vi "Calculate Target Pose.vi"(6 "Distance to target (in)":dbl=36.0, 8 "Robot Calibration Cluster":T1={"Camera Height on robot (in)"=34.5, "Camera Angle on the robot (deg)"=28.3, "Camera FOV Top to Bottom View Angle (deg)"=0.946, "Target size (in)"=6.5, "Distance to front of bumper (in)"=9.75, "Focal Length (mm)"=10.0} {"Focal Length (mm)" format="%#_13g"; "Distance to front of bumper (in)" format="%#_13g"; "Target size (in)" format="%#_13g"; "Camera FOV Top to Bottom View Angle (deg)" format="%#_13g"; "Camera Angle on the robot (deg)" format="%#_13g"; "Camera Height on robot (in)" format="%#_13g"}, 9 "Camera Resolution":T2={"Camera Resolution W (pixels)"=800.0, "Camera Resolution H (pixels)"=600.0}, 10 "Corners":cluster{"X":dbl, "Y":dbl}[](array[cluster])=[{"X"=420.0, "Y"=290.0}, {"X"=480.0, "Y"=290.0}, {"X"=420.0, "Y"=350.0}, {"X"=480.0, "Y"=350.0}], 11 "Target Center":cluster{"X":dbl, "Y":dbl}) -> (1 "Target Roll (deg)":dbl, 2 "Target Pitch (deg)":dbl, 3 "Target Yaw (deg)":dbl)   [LabVIEW 2023]
uses:
  Camera Info.ctl
panel:
  out "3D Position (inches)":cluster{"X":dbl, "Y":dbl, "Z":dbl}
  out "Z'":dbl
  out "Y'":dbl
  out "Z (in)":dbl=36.0
  out "Y (in)":dbl
  out "X (in)":dbl
  out "Theta y (deg)":dbl
  out "Theta x (deg)":dbl
  out "Focal length in pixels":dbl
  out "Sensor height (mm)":dbl
  out "Sensor width (mm)":dbl
  in  "Sensor pixel size (µm)":dbl=3.0
  # "Bottom Left"
  # "Bottom Right"
  # "Top Right"
  # "Top Left"
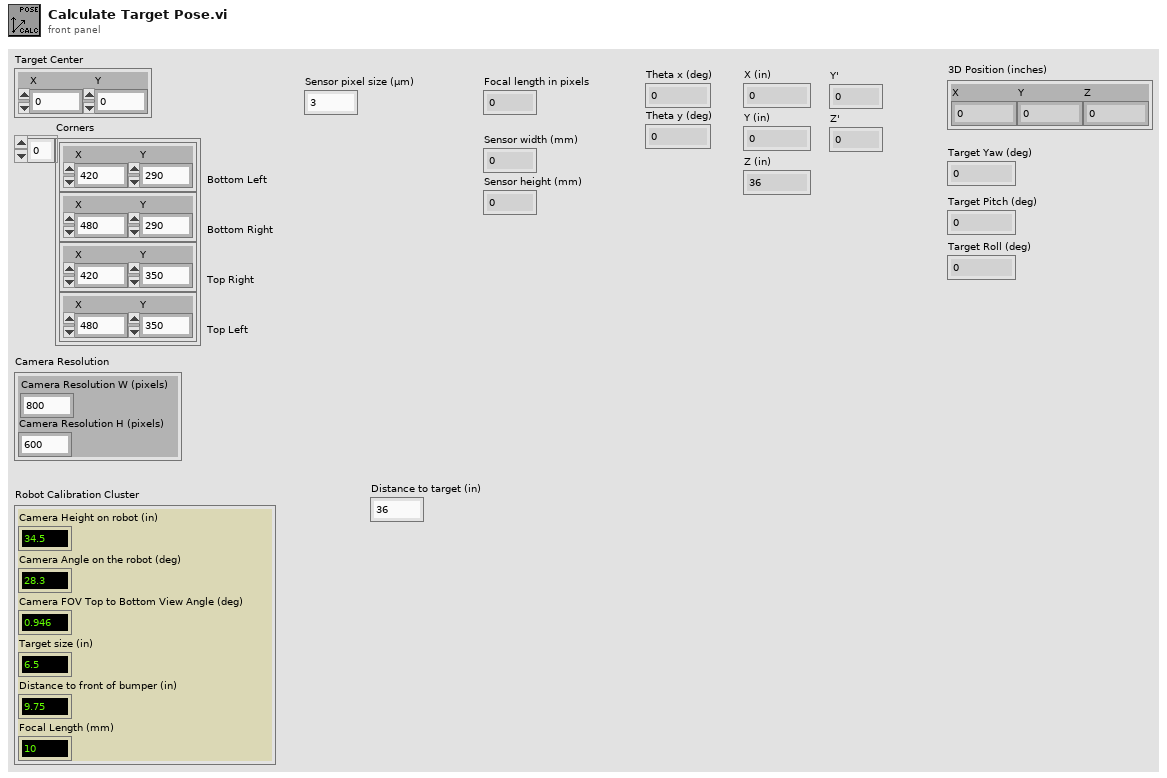
[diagram p1: front panel]
types:
  T1 = typedef "Camera Info.ctl" = cluster{"Camera Height on robot (in)":dbl, "Camera Angle on the robot (deg)":dbl, "Camera FOV Top to Bottom View Angle (deg)":dbl, "Target size (in)":dbl, "Distance to front of bumper (in)":dbl, "Focal Length (mm)":dbl}
  T2 = cluster{"Camera Resolution W (pixels)":dbl, "Camera Resolution H (pixels)":dbl}
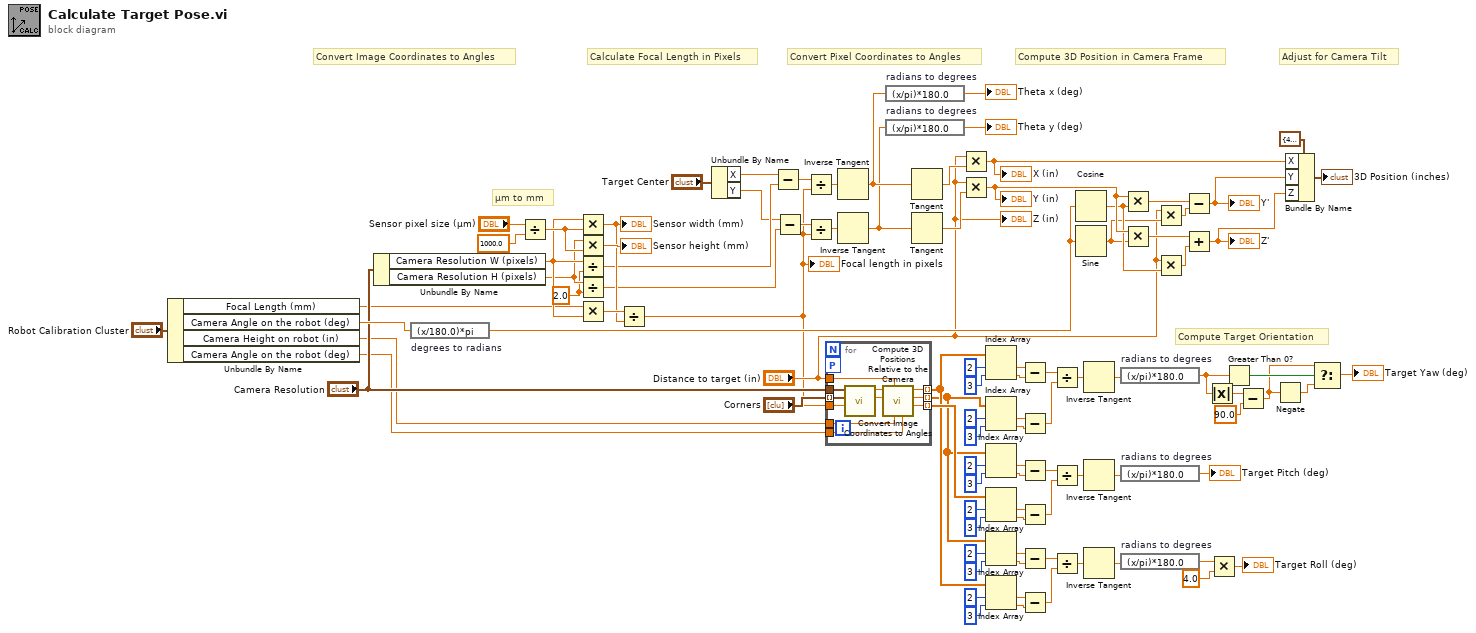
[diagram p0: block diagram]
diagram:
  w65 = 2.0 ("y")
  # "Compute Target Orientation"
  # "Adjust for Camera Tilt"
  # "Compute 3D Position in Camera Frame"
  # "Convert Pixel Coordinates to Angles"
  # "Calculate Focal Length in Pixels"
  # "µm to mm"
  # "Convert Image Coordinates to Angles"
  n1 = Unbundle By Name("Robot Calibration Cluster") -> ("Focal Length (mm)"=w2:dbl, "Camera Angle on the robot (deg)"=w61:dbl, "Camera Height on robot (in)"=w54:dbl, "Camera Angle on the robot (deg)"=w53:dbl)
  n2 = Unbundle By Name("Camera Resolution") -> ("Camera Resolution W (pixels)"=w67:dbl, "Camera Resolution H (pixels)"=w66:dbl)
  n3 = expression code="(x/180.0)*pi" "degrees to radians"(w61) -> (w73:dbl)
  n4 = Divide(x="Sensor pixel size (µm)", y=1000.0) -> (x/y=w94:dbl)
  n5 = Multiply(x=w67, y=w94) -> (x*y=w91:dbl)
  "Sensor width (mm)" <- w91
  n6 = Multiply(x=w66, y=w94) -> (x*y=→"Sensor height (mm)":dbl)
  n7 = Divide(x=w67, y=w65) -> (x/y=w64:dbl)
  n8 = Divide(x=w66, y=w65) -> (x/y=w63:dbl)
  n9 = Multiply(x=w2, y=w67) -> (x*y=w92:dbl)
  n10 = Divide(x=w92, y=w91) -> (x/y=w1:dbl)
  "Focal length in pixels" <- w1
  n11 = Unbundle By Name("Target Center") -> ("X"=w59:dbl, "Y"=w58:dbl)
  n12 = Subtract(x=w59, y=w64) -> (x-y=w90:dbl)
  n13 = Subtract(x=w58, y=w63) -> (x-y=w89:dbl)
  n14 = Divide(x=w90, y=w1) -> (x/y=w88:dbl)
  n15 = Divide(x=w89, y=w1) -> (x/y=w87:dbl)
  n16 = for {
    tunnel: "Camera Resolution" -> [w107]
    tunnel: w1 -> [w106]
    tunnel: "Corners" -> [w105] mode=indexing
    tunnel: "Distance to target (in)" -> [w104]
    tunnel: [w103] -> w14 mode=indexing
    tunnel: [w102] -> w10 mode=indexing
    tunnel: [w101] -> w27 mode=indexing
    tunnel: w54 -> [w100]
    tunnel: w53 -> [w99]
    workers-P: _ -> [_]
    n17 = call "Convert Image Coordinates to Angles.vi"("Focal length in pixels"=w106, "Corner"=w105, "Camera Resolution"=w107) -> ("Thata Y"=w97:dbl, "Thata Z"=w98:dbl)  [unwired: 7 in]
    n18 = call "Compute 3D Positions Relative to the Camera.vi"("Camera Angle on the robot (deg)"=w99, "Camera Height on robot (in)"=w100, "Distance to target (in)"=w104, "Thata Y"=w97, "Thata Z"=w98) -> ("Z Corrected"=w101:dbl, "Y Corrected"=w102:dbl, "X (in)"=w103:dbl)  [unwired: 4 in]
  }
  n19 = Inverse Tangent(1:w88) -> (0:w82:dbl)
  n20 = Inverse Tangent(1:w87) -> (0:w81:dbl)
  n21 = expression code="(x/pi)*180.0" "radians to degrees"(w82) -> (→"Theta x (deg)":dbl)
  n22 = expression code="(x/pi)*180.0" "radians to degrees"(w81) -> (→"Theta y (deg)":dbl)
  n23 = Tangent(1:w82) -> (0:w85:dbl)
  n24 = Tangent(1:w81) -> (0:w83:dbl)
  n25 = Multiply(x="Distance to target (in)", y=w85) -> (x*y=w70:dbl)
  "X (in)" <- w70
  n26 = Multiply(x="Distance to target (in)", y=w83) -> (x*y=w80:dbl)
  "Y (in)" <- w80
  n27 = Index Array(array=w14, index #1=2 ("index"), index #2=3 ("index")) -> (element #1=w50:dbl, element #2=w49:dbl)
  n28 = Index Array(array=w10, index #1=2 ("index"), index #2=3 ("index")) -> (element #1=w47:dbl, element #2=w48:dbl)
  n29 = Index Array(array=w10, index #1=2 ("index"), index #2=3 ("index")) -> (element #1=w31:dbl, element #2=w32:dbl)
  n30 = Index Array(array=w27, index #1=2 ("index"), index #2=3 ("index")) -> (element #1=w34:dbl, element #2=w33:dbl)
  n31 = Index Array(array=w10, index #1=2 ("index"), index #2=3 ("index")) -> (element #1=w24:dbl, element #2=w23:dbl)
  n32 = Index Array(array=w14, index #1=2 ("index"), index #2=3 ("index")) -> (element #1=w21:dbl, element #2=w22:dbl)
  n33 = Subtract(x=w50, y=w49) -> (x-y=w44:dbl)
  n34 = Subtract(x=w47, y=w48) -> (x-y=w43:dbl)
  n35 = Subtract(x=w31, y=w32) -> (x-y=w37:dbl)
  n36 = Subtract(x=w34, y=w33) -> (x-y=w38:dbl)
  n37 = Subtract(x=w24, y=w23) -> (x-y=w18:dbl)
  n38 = Subtract(x=w21, y=w22) -> (x-y=w17:dbl)
  n39 = Divide(x=w44, y=w43) -> (x/y=w42:dbl)
  n40 = Divide(x=w37, y=w38) -> (x/y=w39:dbl)
  n41 = Divide(x=w18, y=w17) -> (x/y=w16:dbl)
  n42 = Cosine(x=w73) -> (cos(x)=w75:dbl)
  n43 = Sine(x=w73) -> (sin(x)=w74:dbl)
  n44 = Inverse Tangent(1:w42) -> (0:w41:dbl)
  n45 = Inverse Tangent(1:w39) -> (0:w40:dbl)
  n46 = Inverse Tangent(1:w16) -> (0:w15:dbl)
  n47 = expression code="(x/pi)*180.0" "radians to degrees"(w41) -> (w7:dbl)
  n48 = expression code="(x/pi)*180.0" "radians to degrees"(w40) -> (→"Target Pitch (deg)":dbl)
  n49 = expression code="(x/pi)*180.0" "radians to degrees"(w15) -> (w12:dbl)
  n50 = Multiply(x=w80, y=w75) -> (x*y=w79:dbl)
  n51 = Multiply(x=w80, y=w74) -> (x*y=w77:dbl)
  n52 = Multiply(x="Distance to target (in)", y=w74) -> (x*y=w78:dbl)
  n53 = Multiply(x="Distance to target (in)", y=w75) -> (x*y=w76:dbl)
  n54 = Subtract(x=w79, y=w78) -> (x-y=w69:dbl)
  "Y'" <- w69
  n55 = Add(x=w77, y=w76) -> (x+y=w68:dbl)
  "Z'" <- w68
  n56 = Absolute Value(x=w7) -> (abs(x)=w8:dbl)
  n57 = Multiply(x=w12, y=4.0) -> (x*y=→"Target Roll (deg)":dbl)
  n58 = Greater Than 0?(x=w7) -> (x > 0?=w6:bool)
  n59 = Subtract(x=w8, y=90.0) -> (x-y=w5:dbl)
  n60 = Negate(x=w5) -> (-x=w4:dbl)
  n61 = Bundle By Name(cluster=cluster{"X":dbl, "Y":dbl, "Z":dbl} {"X"=420.0, "Y"=290.0, "Z"=0.0} ("3D Position (inches)"), "X"=w70, "Y"=w69, "Z"=w68) -> (→"3D Position (inches)":cluster{"X":dbl, "Y":dbl, "Z":dbl})
  n62 = Select(t=w5, s=w6, f=w4) -> (s? t:f=→"Target Yaw (deg)":dbl)
  "Z (in)" <- "Distance to target (in)"
